vi "DDS9959 IO Update.vi"(4 "error in (no error)":errorcluster, 7 "VISA resource name":refnum<visa-resource-name>) -> (0 "error out":errorcluster, 3 "VISA resource name out":refnum<visa-resource-name>)   [LabVIEW 2012]
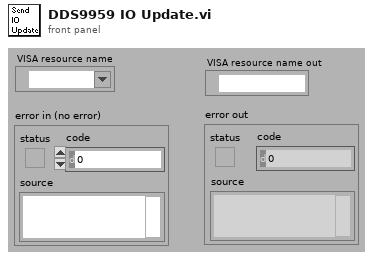
[diagram p1: front panel]
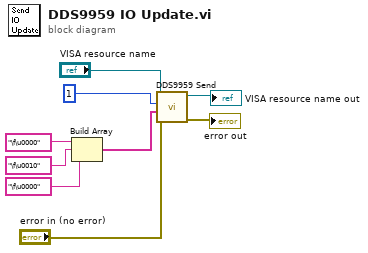
[diagram p0: block diagram]
diagram:
  n1 = Build Array("\f\u0000", "\f\u0010", "\f\u0000") -> (w1:string[])
  n2 = call "DDS9959 Send.vi"("error in (no error)"="error in (no error)", "Output Array"=w1, "USB Out Endpoint"=i16 1, "VISA resource name"="VISA resource name") -> ("error out"=→"error out":errorcluster, "VISA resource name"=→"VISA resource name out":refnum<visa-resource-name>)  [unwired: 6 in]
